vi "DetectEdge(Analog).vi"(5 "EdgeType":enum16{"Rising", "Falling"}(ring), 7 "Level(Voltage)":dbl=3.0 format="%#_13g", 10 "Voltage":dbl) -> (2 "DetectedEdge":bool)   [LabVIEW 2020]
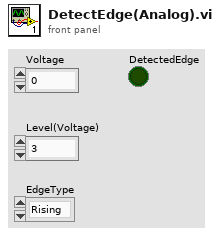
[diagram p1: front panel]
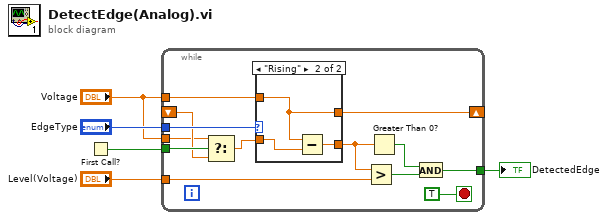
[diagram p0: block diagram]
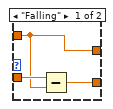
[diagram p2: hidden frame]
diagram:
  n1 = First Call?() -> (First Call?: T/F=w2:bool)
  n2 = while {
    shift-right: [w12] -> _
    shift-left: _ -> [w8]
    tunnel: "Level(Voltage)" -> [w14]
    tunnel: [w17] -> w4
    tunnel: "EdgeType" -> [w11]
    tunnel: "Voltage" -> [w10]
    tunnel: w2 -> [w9]
    tunnel: "Voltage" -> [w6]
    stop <- TRUE stop-if-true
    n3 = Select(t=w6, s=w9, f=w8) -> (s? t:f=w7:dbl)
    n4 = case shown="\"Rising\"" w11 {
      tunnel: [w21 w24] -> w13
      tunnel: w7 -> [w20 w23]
      tunnel: [w19 w22] -> w12
      tunnel: w10 -> [w19 w22]
      frame "Falling" {
        n5 = Subtract(x=w20, y=w19) -> (x-y=w21:dbl)
      }
      frame "Rising" {
        n6 = Subtract(x=w22, y=w23) -> (x-y=w24:dbl)
      }
    }
    n7 = Greater?(x=w13, y=w14) -> (0:w15:bool)
    n8 = Greater Than 0?(x=w13) -> (x > 0?=w16:bool)
    n9 = And(x=w16, y=w15) -> (x .and. y?=w17:bool)
  }
  "DetectedEdge" <- w4
